vi "saveViPos.vi"(11 "error in (no error)":errorcluster) -> (3 "error out":errorcluster)   [LabVIEW 2016]
uses:
  <vilib>/Utility/file.llb/Write Delimited Spreadsheet (I64).vi
  <vilib>/Utility/file.llb/Read Delimited Spreadsheet (DBL).vi
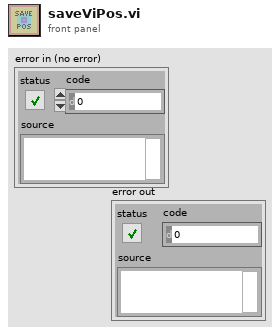
[diagram p1: front panel]
types:
  T1 = typedef "LVRectTypeDef.ctl" = cluster{"Left":i16, "Top":i16, "Right":i16, "Bottom":i16}
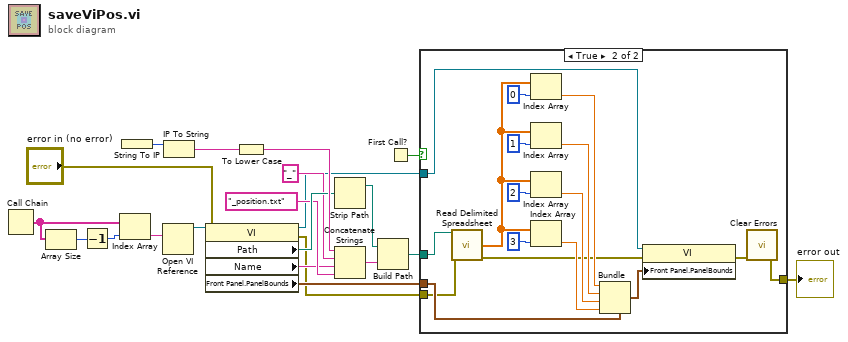
[diagram p0: block diagram]
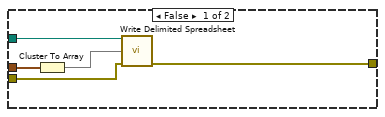
[diagram p2: hidden frame]
diagram:
  n1 = Call Chain() -> (call chain=w10:string[])
  n2 = Array Size(array=w10) -> (size(s)=w9:i32)
  n3 = Decrement(x=w9) -> (x-1=w8:i32)
  n4 = Index Array(array=w10, index=w8) -> (element=w7:string)
  n5 = String To IP() -> (0:w19:u32)  [unwired: 1 in]
  n6 = Open VI Reference(vi path=w7) -> (vi reference=w6:refnum<vi>)  [unwired: 5 in, 1 out]
  n7 = IP To String(2:w19) -> (0:w18:string)  [unwired: 1 in]
  n8 = property class="VI"(reference=w6, error in="error in (no error)") -> (reference out=w4:refnum<vi>, error out=w2:errorcluster, "Path"=w15:path, "Name"=w12:string, "Front Panel.PanelBounds"=w5:T1)
  n9 = To Lower Case(string=w18) -> (all lower case string=w17:string)
  n10 = Strip Path(path=w15) -> (stripped path=w21:path)  [unwired: 1 out]
  n11 = Concatenate Strings(w17, "_" ("string"), w12, "_position.txt" ("name or relative path")) -> (w16:string)
  n12 = Build Path(base path=w21, name or relative path=w16) -> (appended path=w20:path)
  n13 = First Call?() -> (First Call?: T/F=w11:bool)
  n14 = case shown="True" w11 {
    tunnel: w20 -> [w26 w43]
    tunnel: w5 -> [w24 w42]
    tunnel: w4 -> [_ w29]
    tunnel: w2 -> [w23 w28]
    tunnel: [w22 w27] -> w1
    frame False {
      n15 = Cluster To Array(cluster=w24) -> (array=w25:i16[])
      n16 = call-poly <vilib>:"Write Delimited Spreadsheet.vi"("file path (dialog if empty)"=w26, "1D data"=w25, "error in (no error)"=w23) -> ("error out"=w22:errorcluster)  [unwired: 11 in, 1 out]
    }
    frame True {
      n17 = call-poly <vilib>:"Read Delimited Spreadsheet.vi"("file path (dialog if empty)"=w43, "error in (no error)"=w28) -> ("first row"=w40:dbl[], "error out"=w31:errorcluster)  [unwired: 8 in, 4 out]
      n18 = Index Array(array=w40, index=0) -> (element=w38:dbl)
      n19 = Index Array(array=w40, index=1) -> (element=w37:dbl)
      n20 = Index Array(array=w40, index=2) -> (element=w36:dbl)
      n21 = Index Array(array=w40, index=3) -> (element=w35:dbl)
      n22 = Bundle(cluster=w42, "Left"=w38, "Top"=w37, "Right"=w36, "Bottom"=w35) -> (w41:T1)
      n23 = property class="VI"(reference=w29, error in=w31, "Front Panel.PanelBounds"=w41) -> (error out=w30:errorcluster)  [unwired: 1 out]
      n24 = call <vilib>:"Clear Errors.vi"("error in (no error)"=w30) -> ("error out"=w27:errorcluster)  [unwired: 5 in, 1 out]
    }
  }
  "error out" <- w1
